vi "Create.vi"(5 "Test Suite in":refnum<class "Test Suite.lvclass">, 6 "Hostname (\"localhost\")":string="localhost", 7 "Timestamp":timestamp, 8 "error in (no error)":errorcluster, 9 "Id":i32, 10 "Name":string, 11 "Package":string) -> (0 "error out":errorcluster, 3 "Test Suite":refnum<class "Test Suite.lvclass">)   [LabVIEW 2013, in "JUnit XML.lvlib" / "Test Suite.lvclass"]
uses:
  Test Suite.lvclass
  Test Suite.lvclass/Test Suite.ctl
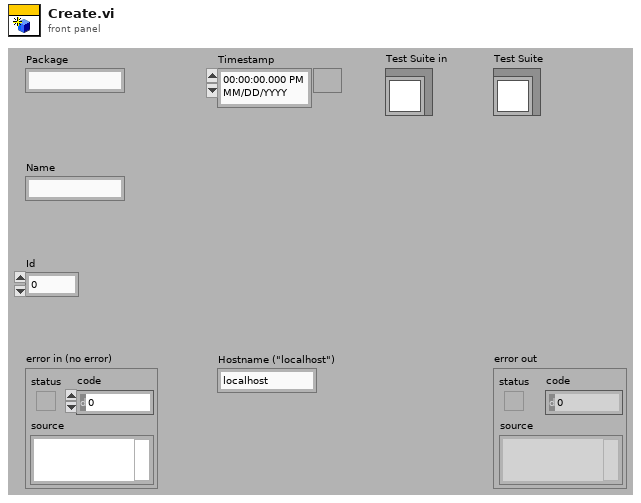
[diagram p1: front panel]
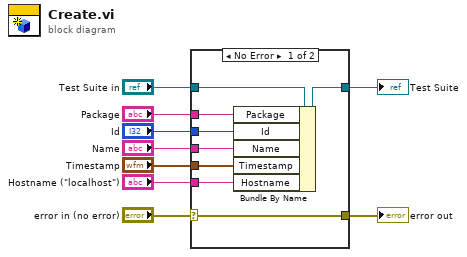
[diagram p0: block diagram]
diagram:
  n1 = case shown="No Error" "error in (no error)" {
    selector: "error in (no error)" -> [w17 w19]
    tunnel: [w17 w19] -> w8
    tunnel: [w15 w18] -> w6
    tunnel: "Test Suite in" -> [w16 w18]
    tunnel: "Package" -> [w14 _]
    tunnel: "Id" -> [w13 _]
    tunnel: "Name" -> [w12 _]
    tunnel: "Timestamp" -> [w11 _]
    tunnel: "Hostname (\"localhost\")" -> [w10 _]
    frame No Error {
      n2 = Bundle By Name(cluster=w16, "Package"=w14, "Id"=w13, "Name"=w12, "Timestamp"=w11, "Hostname"=w10) -> (w15:refnum<class "Test Suite.lvclass">)
    }
    frame Error {
    }
  }
  "error out" <- w8
  "Test Suite" <- w6
